vi "OPCUA.vi"(8 "error In":errorcluster, 9 "Ignition FGVname":string="Ignition Ref", 10 "Ignition Folder names":string[](array[string]), 11 "Sequence Context In":refnum<k7>) -> (0 "error out":errorcluster, 2 "Connect?":bool, 3 "subscription ID":T1)   [LabVIEW 2021, in "OPCUA.lvlib"]
doc: "Use this template to build a simple state machine design pattern. Each state executes code and determines which state to transition to."
uses:
  OPCUA.lvlib
  Controls/Tester Rx.ctl
  Controls/Tester Tx.ctl
  <vilib>/OPCUA/controls/Subscription ID.ctl
  Controls/Local Dataset.ctl
  Controls/State.ctl
  <vilib>/OPCUA/controls/Write Status.ctl
  02c02d1d-dd3a-4c13-a0d3-6ac730eac6fc.vi
  <vilib>/OPCUA/client/Multiple Write Variant.vi
  <vilib>/OPCUA/NI OPC UA Client.lvlib
panel:
  out "Timeout":bool
  out "Note":string
  out "Station":string
  in  "Tester Tx":T2
  out "Tester Rx":T3
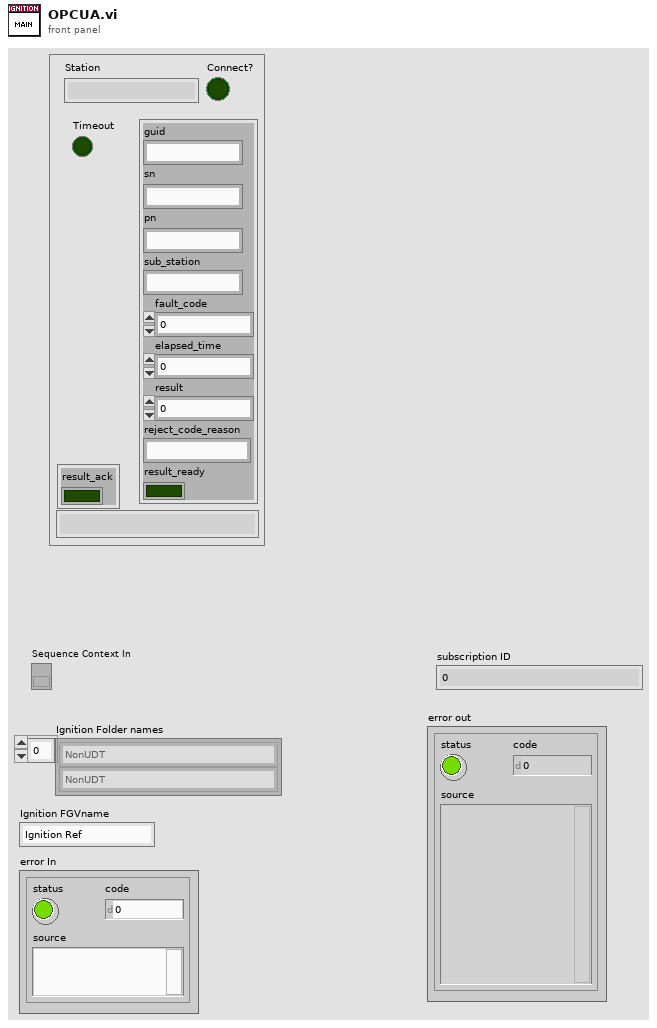
[diagram p1: front panel]
types:
  T1 = typedef "Subscription ID.ctl" = u32
  T2 = typedef "OPCUA.lvlib/Tester Tx.ctl" = cluster{"guid":string, "sn":string, "pn":string, "sub_station":string, "fault_code":i32, "elapsed_time":i32, "result":i32, "reject_code_reason":string, "result_ready":bool}
  T3 = typedef "OPCUA.lvlib/Tester Rx.ctl" = cluster{"result_ack":bool}
  T4 = typedef "OPCUA.lvlib/State.ctl" = enum16{"Initialize", "Set Dataset", "Wait for Event", "Stop", "Exit"}
  T5 = typedef "OPCUA.lvlib/Local Dataset.ctl" = cluster{"NodeIDs":string[][], "Tester Tx":refnum<vi>, "Tester Rx":refnum<vi>}
  T6 = typedef "OPC UA Client Refnum.ctl" = refnum<k21>
  T7 = typedef "TestStand - Status Monitor.ctl" = cluster{"Sequence Context":refnum<k7>, "Execution":refnum<k7>, "Termination Monitor":refnum<k7>}
  T8 = typedef "Subscription Data Change.ctl" = cluster{"node ID":T9, " value":variant, "timestamp":timestamp, "data type":T10, "status code":T11}
  T9 = typedef "NodeId.ctl" = string
  T10 = typedef "Data Type.ctl" = u16
  T11 = typedef "OPC UA StatusCode.ctl" = u32
  T12 = typedef "Ignition.lvlib/Tester Rx.ctl" = cluster{"result_ack":bool}
  T13 = typedef "Write Status.ctl" = u32
  T14 = typedef "Write Variant Request.ctl" = cluster{"node ID":T9, "value":variant, "timestamp (current time)":timestamp, "node status":T13}
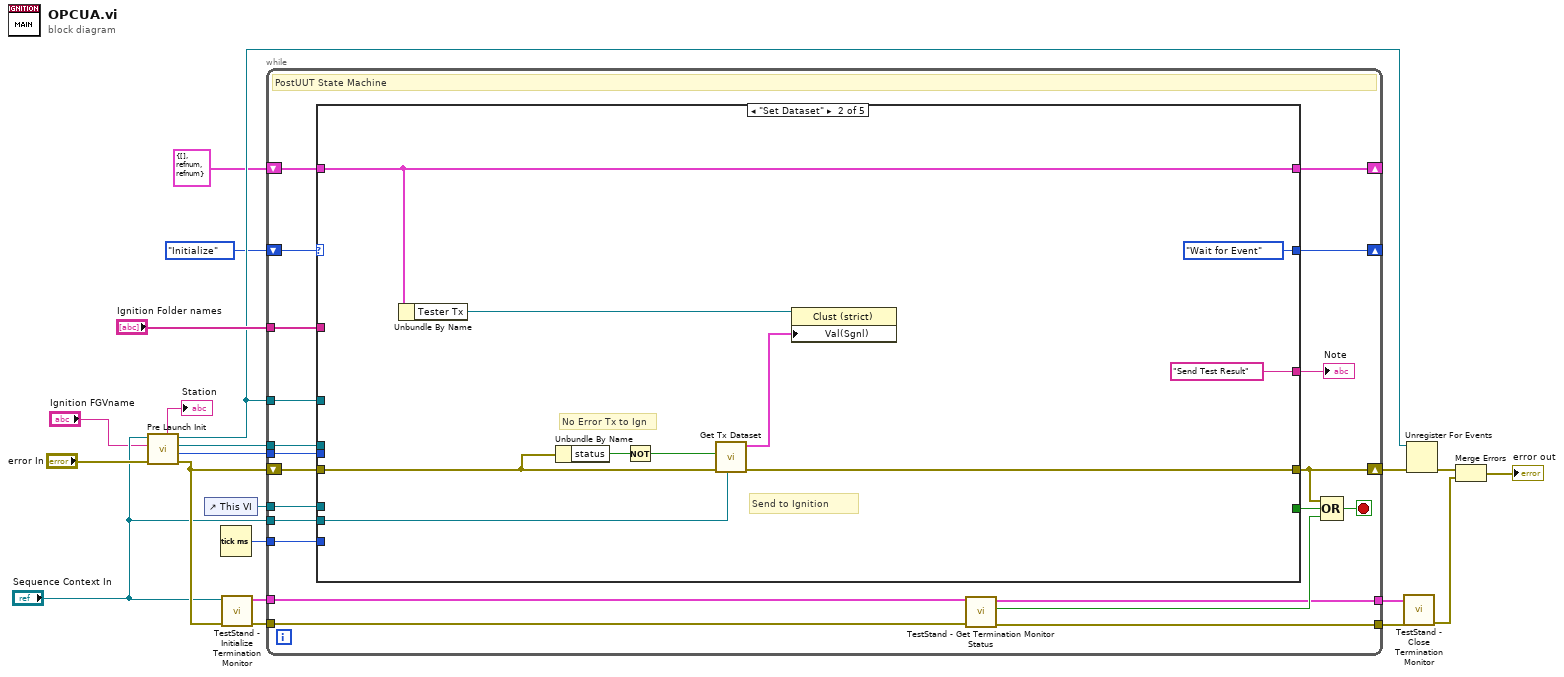
[diagram p0: block diagram]
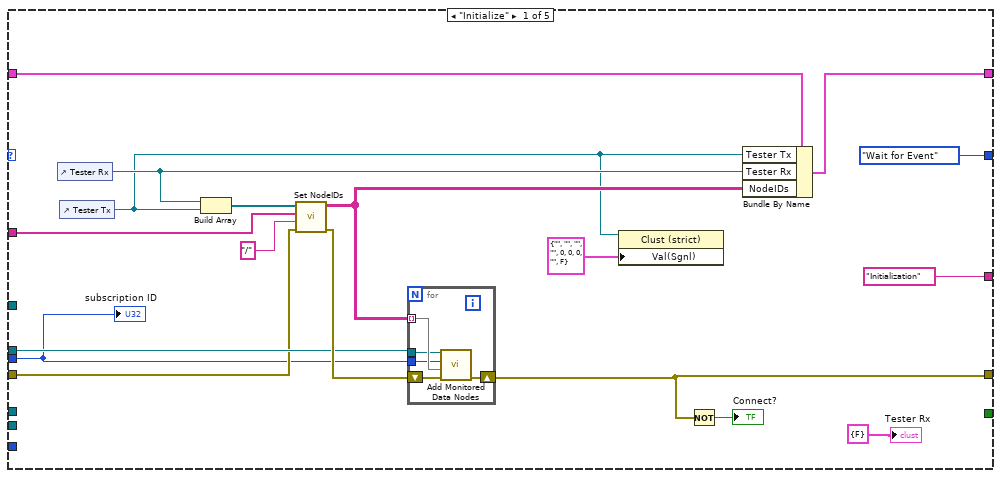
[diagram p2: hidden frame]
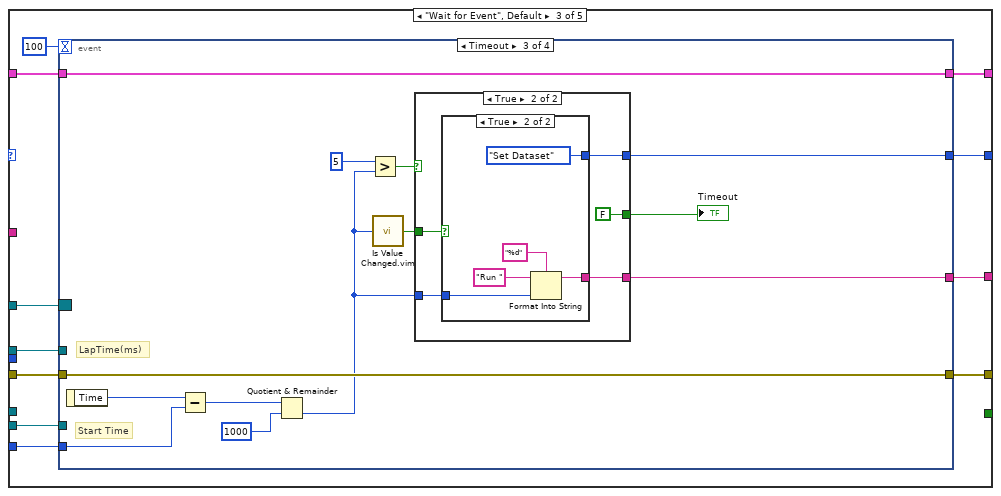
[diagram p3: hidden frame]
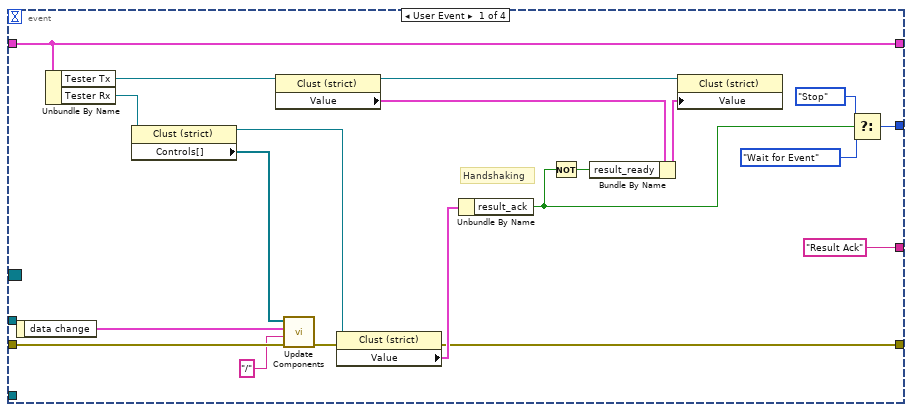
[diagram p4: hidden frame]
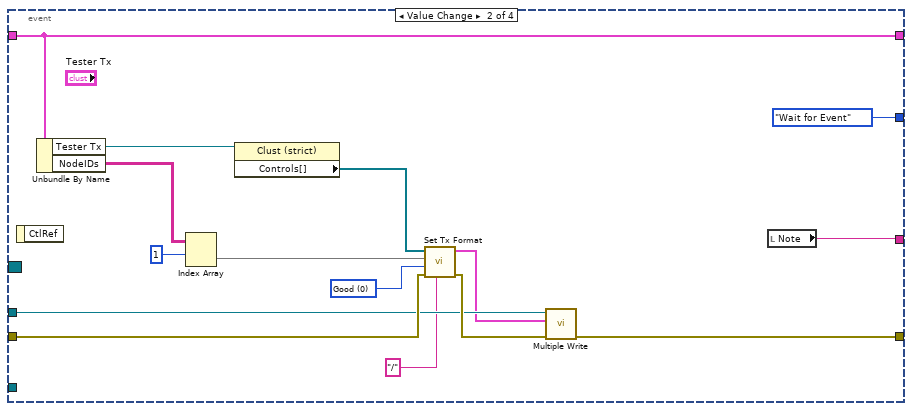
[diagram p5: hidden frame]
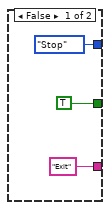
[diagram p6: hidden frame]
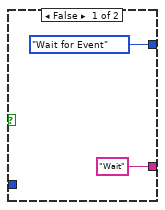
[diagram p7: hidden frame]
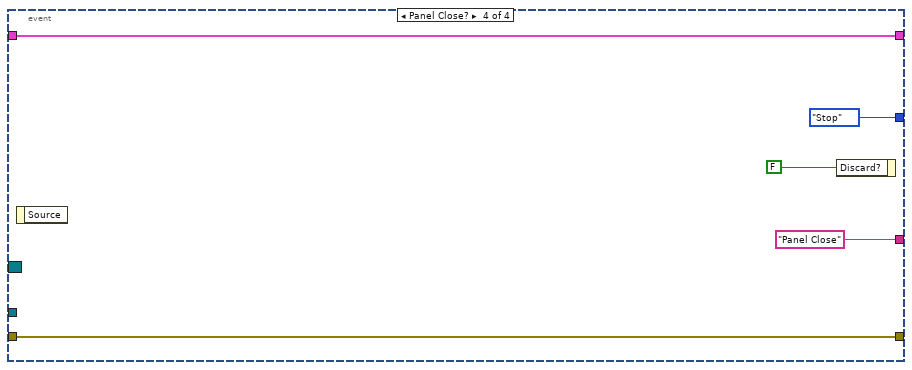
[diagram p8: hidden frame]
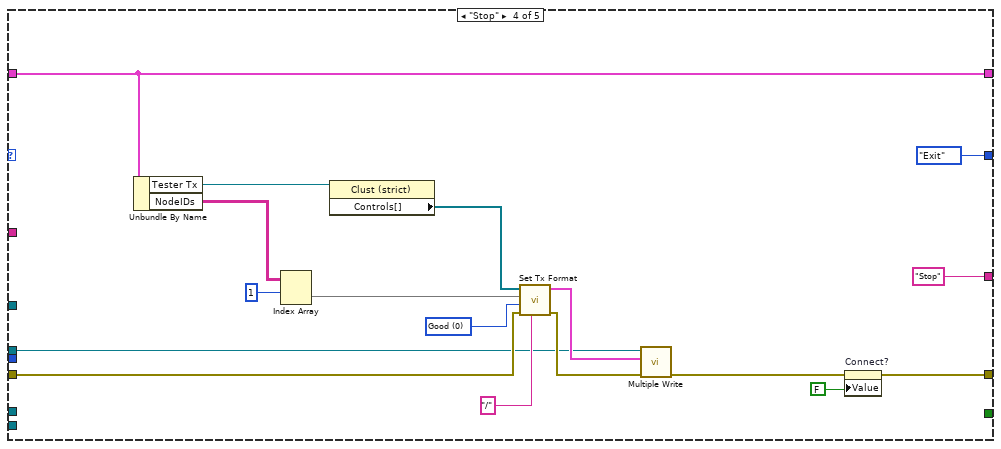
[diagram p9: hidden frame]
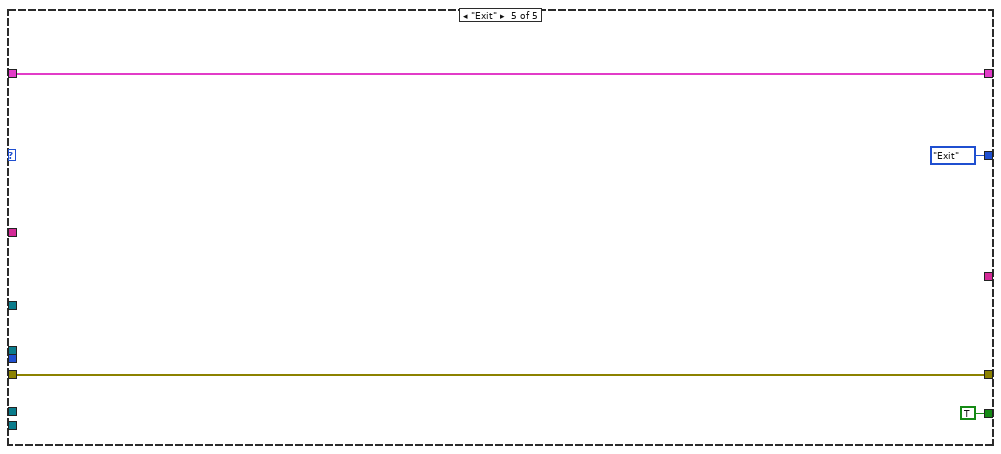
[diagram p10: hidden frame]
diagram:
  n1 = call "Pre Launch Init.vi"("error in"="error In", "FGV Name"="Ignition FGVname", "Sequence Context In"="Sequence Context In") -> ("error out"=w13:errorcluster, "OPC subscriptID"=w12:T1, "OPC Client ref"=w11:T6, "Event Registration Refnum"=w4:refnum<event-registration>, "Station"=→"Station":string)  [unwired: 4 in]
  n2 = control-ref of="This VI"() -> (w7:refnum<vi>)
  n3 = Tick Count (ms)() -> (millisecond timer value=w10:u32)
  n4 = call <vilib>:"TestStand - Initialize Termination Monitor.vi"("error in (no error)"=w13, "Sequence Context In"="Sequence Context In") -> ("error out"=w19:errorcluster, "Status Monitor Out"=w20:T7)  [unwired: 8 in]
  n5 = while {
    shift-right: [w41] -> _
    shift-left: State."Initialize" ("States") -> [w42]
    shift-right: [w24] -> _
    shift-left: T5 {"NodeIDs"=[], "Tester Tx"=refnum, "Tester Rx"=refnum} ("Data") -> [w40]
    shift-right: [w33] -> w6
    shift-left: w13 -> [w39]
    tunnel: "Ignition Folder names" -> [w38]
    tunnel: w11 -> [w37]
    tunnel: w12 -> [w36]
    tunnel: w4 -> [w35]
    tunnel: w20 -> [w34]
    tunnel: [w29] -> w17
    tunnel: w19 -> [w28]
    tunnel: [w27] -> w16
    tunnel: "Sequence Context In" -> [w26]
    tunnel: w10 -> [w25]
    tunnel: w7 -> [w22]
    stop <- w30 stop-if-true
    # "PostUUT State Machine"
    n6 = case shown="\"Set Dataset\"" w42 {
      tunnel: [State."Wait for Event" ("States") State."Wait for Event" ("States") w86 State."Exit" ("States") State."Exit" ("States")] -> w41
      tunnel: [_ _ _ _ TRUE ("Stop Loop?")] -> w32
      tunnel: w40 -> [w60 w75 w85 w160 w175]
      tunnel: [w52 w75 w80 w160 w175] -> w24
      tunnel: w39 -> [w55 w69 w83 w159 w174]
      tunnel: [w50 w73 w84 w169 w174] -> w33
      tunnel: w38 -> [w57 _ _ _ _]
      tunnel: w37 -> [w56 _ w81 w158 _]
      tunnel: w36 -> [w54 _ _ _ _]
      tunnel: w35 -> [_ _ w82 _ _]
      tunnel: w26 -> [_ w72 w79 _ _]
      tunnel: w25 -> [_ _ w77 _ _]
      tunnel: ["Initialization" ("Note") "Send Test Result" ("Note") w76 "Stop" ("Note") _] -> w23
      tunnel: w22 -> [_ _ _ _ _]
      frame "Initialize" {
        # "Initialize - Initialize the application."
        n7 = control-ref of="Tester Rx"() -> (w47:refnum<vi>)
        n8 = control-ref of="Tester Tx"() -> (w43:refnum<vi>)
        n9 = Build Array(w47, w43) -> (w49:refnum<vi>[])
        n10 = call "Set NodeIDs.vi"("error in (no error)"=w55, "Deliminated Char"="/", "Folder names"=w57, "Control Refs"=w49) -> ("error out"=w59:errorcluster, "NodeIDs"=w58:string[][])  [unwired: 6 in]
        n11 = for {
          shift-right: [w65] -> w50
          shift-left: w59 -> [w64]
          tunnel: w58 -> [w63] mode=indexing
          tunnel: w56 -> [w62]
          tunnel: w54 -> [w61]
          n12 = call <vilib>:"Add Monitored Data Nodes.vi"("error in (no error)"=w64, "node IDs"=w63, "subscription ID in"=w61, "OPC UA client refnum in"=w62) -> ("error out"=w65:errorcluster)  [unwired: 4 in, 3 out]
        }
        n13 = property class="Clust (strict)"(reference=w43, "Val(Sgnl)"=T2 {"guid"="", "sn"="", "pn"="", "sub_station"="", "fault_code"=0, "elapsed_time"=0, "result"=0, "reject_code_reason"="", "result_ready"=FALSE} ("Tester Tx")) -> ()  [unwired: 1 in, 2 out]
        n14 = Not(x=w50) -> (.not. x?=→"Connect?":bool)
        n15 = Bundle By Name(cluster=w60, "Tester Tx"=w43, "Tester Rx"=w47, "NodeIDs"=w58) -> (w52:T5)
        "subscription ID" <- w54
        "Tester Rx" <- T3 {"result_ack"=FALSE} ("Tester Rx")
      }
      frame "Set Dataset" {
        # "No Error Tx to Ign"
        # "Send to Ignition"
        n16 = Unbundle By Name(w75) -> ("Tester Tx"=w71:refnum<vi>)
        n17 = Unbundle By Name(w69) -> ("status"=w68:bool)
        n18 = Not(x=w68) -> (.not. x?=w67:bool)
        n19 = call "Get Tx Dataset.vi"("Sequence Context In"=w72, "error in"=w69, "result_ready"=w67) -> ("error out"=w73:errorcluster, "Tester Tx"=w70:T2)  [unwired: 7 in]
        n20 = property class="Clust (strict)"(reference=w71, "Val(Sgnl)"=w70) -> ()  [unwired: 1 in, 2 out]
      }
      frame "Wait for Event", Default {
        # "Wait for Event - Use an Event Structure to monitor the user interface for events that run different states of the state machine."
        n21 = event shown="[2] Timeout" {
          selector: w82 -> [_ _ _ _]
          dyn-events: _ -> [_ _ _ _]
          timeout: 100 -> [_ _ _ _]
          tunnel: [w100 State."Wait for Event" ("States") w126 State."Stop" ("States")] -> w86
          tunnel: w85 -> [w96 w115 w128 w153]
          tunnel: [w96 w115 w128 w153] -> w80
          tunnel: w83 -> [w106 w121 w132 w151]
          tunnel: [w98 w110 w132 w151] -> w84
          tunnel: w81 -> [_ w116 _ _]
          tunnel: w79 -> [_ _ _ _]
          tunnel: w77 -> [_ _ w133 _]
          tunnel: ["Result Ack" ("Note") w109 w124 "Panel Close" ("Note")] -> w76
          event User Event {
            # "Handshaking"
            n22 = event-data() -> ("data change"=w104:T8[])  [unwired: 1 in]
            n23 = Unbundle By Name(w96) -> ("Tester Tx"=w94:refnum<vi>, "Tester Rx"=w103:refnum<vi>)
            n24 = property class="Clust (strict)"(reference=w103) -> (reference out=w101:refnum<vi>, "Controls[]"=w105:refnum<vi>[])  [unwired: 1 in, 1 out]
            n25 = property class="Clust (strict)"(reference=w94) -> (reference out=w93:refnum<vi>, "Value"=w92:T2)  [unwired: 1 in, 1 out]
            n26 = call "Update Components.vi"("error in (no error)"=w106, "Deliminated Char"="/", "data change"=w104, "Controls"=w105) -> ("error out"=w99:errorcluster)  [unwired: 7 in]
            n27 = property class="Clust (strict)"(reference=w101, error in=w99) -> (error out=w98:errorcluster, "Value"=w102:T12)  [unwired: 1 out]
            n28 = Unbundle By Name(w102) -> ("result_ack"=w90:bool)
            n29 = Not(x=w90) -> (.not. x?=w89:bool)
            n30 = Bundle By Name(cluster=w92, "result_ready"=w89) -> (w91:T2)
            n31 = property class="Clust (strict)"(reference=w93, "Value"=w91) -> ()  [unwired: 1 in, 2 out]
            n32 = Select(t=State."Stop" ("States"), s=w90, f=State."Wait for Event" ("States")) -> (s? t:f=w100:T4)
          }
          event Value Change {
            w120 = T13 0 items=["Good"=0, "Uncertain"=1073741824, "Uncertain_InitialValue"=1083310080, "Uncertain_LastUsableValue"=1083179008, "Uncertain_SensorNotAccurate"=1083375616, "Uncertain_EngineeringUnitsExceeded"=1083441152, "Bad"=2147483648, "Bad_NoCommunication"=2150694912, "Bad_NotReadable"=2151284736, "Bad_NotWritable"=2151350272, "Bad_OutOfRange"=2151415808, "Bad_WaitingForInitialData"=2150760448] ("node status")
            n33 = event-data() -> ()  [unwired: 1 in, 1 out]
            n34 = Unbundle By Name(w115) -> ("Tester Tx"=w111:refnum<vi>, "NodeIDs"=w119:string[][])
            n35 = Index Array(array=w119, index (row)=1) -> (element=w114:string[])  [unwired: 1 in]
            n36 = property class="Clust (strict)"(reference=w111) -> ("Controls[]"=w112:refnum<vi>[])  [unwired: 1 in, 2 out]
            n37 = call "Set Tx Format.vi"("Delimitated Char"="/", "error in (no error)"=w121, "node status"=w120, "NodeIDs"=w114, "Controls"=w112) -> ("error out"=w117:errorcluster, "Dataset"=w113:T14[])  [unwired: 5 in]
            n38 = call-poly <vilib>:"Multiple Write.vi"("error in (no error)"=w117, "requests"=w113, "OPC UA client refnum in"=w116) -> ("error out"=w110:errorcluster)  [unwired: 5 in, 3 out]
            n39 = local read "Note"() -> (w109:string)
          }
          event Timeout {
            # "LapTime(ms)"
            # "Start Time"
            n40 = event-data() -> ("Time"=w134:u32)  [unwired: 1 in]
            n41 = Subtract(x=w134, y=w133) -> (x-y=w131:u32)
            n42 = Quotient & Remainder(x=w131, y=u32 1000) -> (floor(x/y)=w123:u32)  [unwired: 1 out]
            n43 = Greater?(x=u32 5, y=w123) -> (0:w127:bool)
            n44 = call "Is Value Changed.vim"("value"=w123) -> ("changed or first call?"=w125:bool)
            n45 = case shown="True" w127 {
              tunnel: [State."Stop" ("States") w139] -> w126
              tunnel: w125 -> [_ w142]
              tunnel: ["Exit" ("Note") w141] -> w124
              tunnel: w123 -> [_ w140]
              tunnel: [TRUE ("Timeout") FALSE ("Timeout")] -> w122
              frame False {
              }
              frame True {
                n46 = case shown="True" w142 {
                  tunnel: ["Wait" ("Note") w146] -> w141
                  tunnel: w140 -> [_ w148]
                  tunnel: [State."Wait for Event" ("States") State."Set Dataset" ("States")] -> w139
                  frame False {
                  }
                  frame True {
                    n47 = Format Into String(format string="%d", initial string="Run " ("Note"), w148) -> (resulting string=w146:string)  [unwired: 1 in, 1 out]
                  }
                }
              }
            }
            "Timeout" <- w122
          }
          event Panel Close? {
            n48 = event-data() -> ()  [unwired: 1 in, 1 out]
            n49 = event-data("Discard?"=FALSE) -> ()  [unwired: 1 in, 1 out]
          }
        }
      }
      frame "Stop" {
        w162 = T13 0 items=["Good"=0, "Uncertain"=1073741824, "Uncertain_InitialValue"=1083310080, "Uncertain_LastUsableValue"=1083179008, "Uncertain_SensorNotAccurate"=1083375616, "Uncertain_EngineeringUnitsExceeded"=1083441152, "Bad"=2147483648, "Bad_NoCommunication"=2150694912, "Bad_NotReadable"=2151284736, "Bad_NotWritable"=2151350272, "Bad_OutOfRange"=2151415808, "Bad_WaitingForInitialData"=2150760448] ("node status")
        # "Exit - Exit the application."
        n50 = Unbundle By Name(w160) -> ("Tester Tx"=w156:refnum<vi>, "NodeIDs"=w168:string[][])
        n51 = Index Array(array=w168, index (row)=1) -> (element=w166:string[])  [unwired: 1 in]
        n52 = property class="Clust (strict)"(reference=w156) -> ("Controls[]"=w164:refnum<vi>[])  [unwired: 1 in, 2 out]
        n53 = call "Set Tx Format.vi"("Delimitated Char"="/", "error in (no error)"=w159, "node status"=w162, "NodeIDs"=w166, "Controls"=w164) -> ("error out"=w167:errorcluster, "Dataset"=w165:T14[])  [unwired: 5 in]
        n54 = call-poly <vilib>:"Multiple Write.vi"("error in (no error)"=w167, "requests"=w165, "OPC UA client refnum in"=w158) -> ("error out"=w157:errorcluster)  [unwired: 5 in, 3 out]
        n55 = property on="Connect?" class="Bool (strict)"(error in=w157, "Value"=FALSE ("Network")) -> (error out=w169:errorcluster)  [unwired: 1 in, 1 out]
      }
      frame "Exit" {
      }
    }
    "Note" <- w23
    n56 = call <vilib>:"TestStand - Get Termination Monitor Status.vi"("error in (no error)"=w28, "Status Monitor In"=w34) -> ("error out"=w27:errorcluster, "Terminating or Aborting"=w31:bool, "Status Monitor Out"=w29:T7)  [unwired: 7 in]
    n57 = Compound Arithmetic op=OR(w33, w32, w31) -> (w30:bool)
  }
  n58 = call <vilib>:"TestStand - Close Termination Monitor.vi"("error in (no error)"=w16, "Status Monitor In"=w17) -> ("error out"=w15:errorcluster)  [unwired: 9 in]
  n59 = Unregister For Events(event registration refnum=w4, error in=w6) -> (error out=w5:errorcluster)
  n60 = Merge Errors(w5, w15) -> (→"error out":errorcluster)
